vi "PRL Channel Selector Configuration.vi"(8 "Signal Names In":T1, 10 "Get All Signals":bool, 11 "Action":T2(ring)=enum."Get All Signal Names") -> (0 "Signal Names Out":T1)   [LabVIEW 2013, in "PMU Recorder Light.lvlib"]
uses:
  PMU Recorder Light.lvlib
panel:
  out "error out":errorcluster
  in  "error in (no error)":errorcluster
  # "INPUT"
  # "INTERMEDIATE"
  # "OUTPUT"
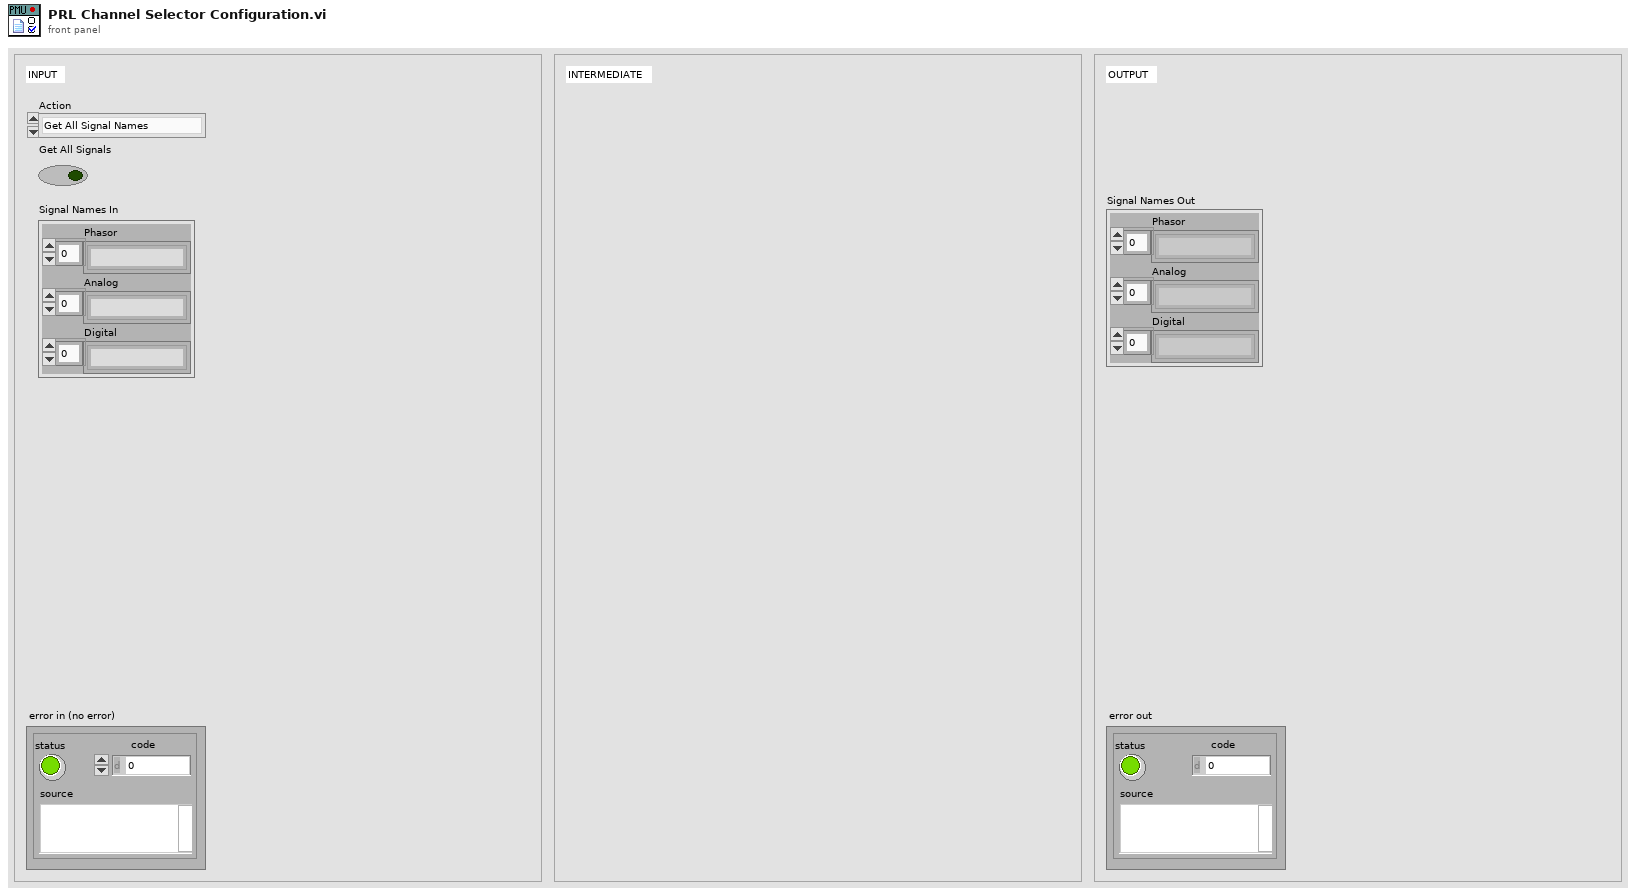
[diagram p1: front panel]
types:
  T1 = cluster{"Phasor":string[], "Analog":string[], "Digital":string[]}
  T2 = enum16{"Filter Signals", "Get All Signal Names", "Select Signals on Name", "Select Frequency Only", "Get Selected Signal Names"}
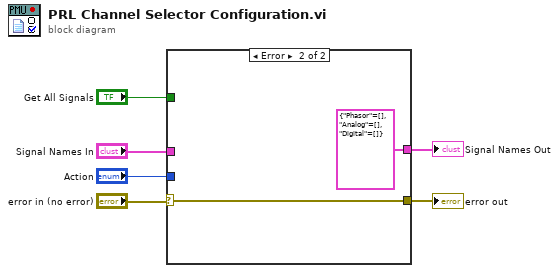
[diagram p0: block diagram]
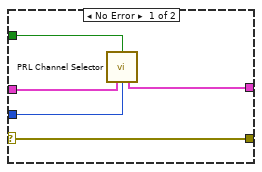
[diagram p2: hidden frame]
diagram:
  n1 = case shown="Error" "error in (no error)" {
    selector: "error in (no error)" -> [w7 w12]
    tunnel: "Action" -> [w11 _]
    tunnel: "Signal Names In" -> [w10 _]
    tunnel: [w9 T1 {"Phasor"=[], "Analog"=[], "Digital"=[]} ("Signal Names Out")] -> w4
    tunnel: "Get All Signals" -> [w8 _]
    tunnel: [w7 w12] -> w1
    frame No Error {
      n2 = call "PRL Channel Selector.vi"("Get All Signals"=w8, "Signal Names In"=w10, "Action"=w11) -> ("Signal Names Out"=w9:T1)  [unwired: 9 in, 3 out]
    }
    frame Error {
    }
  }
  "Signal Names Out" <- w4
  "error out" <- w1
